vi "Write Element of Exp Groups.vi"(8 "error in (no error)":errorcluster, 9 "Experiments_group.lvclass":refnum<class "Experiments_group.lvclass">, 10 "index":i32=-1, 11 "Control-Client in":refnum<class "Control-Client.lvclass">) -> (0 "error out":errorcluster, 3 "Control-Client out":refnum<class "Control-Client.lvclass">)   [LabVIEW 2018, in "Control-Client.lvclass"]
uses:
  Control-Client.lvclass
  Experiments/Experiments_group.lvclass
  Control-Client.lvclass/Control-Client.ctl
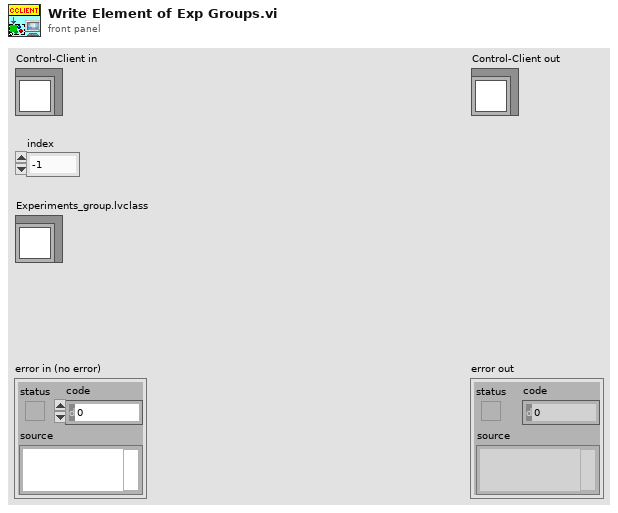
[diagram p1: front panel]
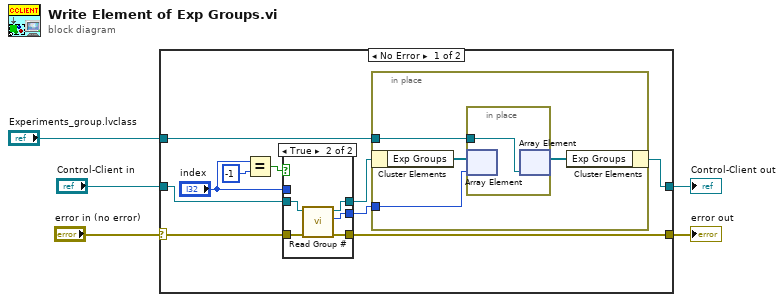
[diagram p0: block diagram]
diagram:
  n1 = case shown="No Error" "error in (no error)" {
    selector: "error in (no error)" -> [w11 w29]
    tunnel: [w12 w29] -> w4
    tunnel: [w7 w30] -> w2
    tunnel: "Control-Client in" -> [w10 w30]
    tunnel: "Experiments_group.lvclass" -> [w8 _]
    frame No Error {
      n2 = Equal?(x="index", y=-1) -> (x = y?=w14:bool)
      n3 = case shown="True" w14 {
        tunnel: [w23 w28] -> w9
        tunnel: "index" -> [w23 _]
        tunnel: [w22 w27] -> w12
        tunnel: w11 -> [w22 w26]
        tunnel: w10 -> [w21 w25]
        tunnel: [w21 w24] -> w6
        frame False {
        }
        frame True {
          n4 = call "Read Group #.vi"("error in (no error)"=w26, "Control-Client in"=w25) -> ("error out"=w27:errorcluster, "Group #"=w28:i32, "Control-Client out"=w24:refnum<class "Control-Client.lvclass">)  [unwired: 7 in]
        }
      }
      n5 = in-place {
        in-place-border: w9 -> [w18]
        in-place-border: w8 -> [w16]
        n6 = in-place-cluster #1(w6) -> ("Exp Groups"=w19:refnum<class "Experiments_group.lvclass">[])
        n7 = in-place {
          in-place-border: w16 -> [w20]
          n8 = in-place-array #2(w19, w18) -> ()  [unwired: 1 out]
          n9 = in-place-array #2(w20) -> (w17:refnum<class "Experiments_group.lvclass">[])  [unwired: 1 out]
        }
        n10 = in-place-cluster #1("Exp Groups"=w17) -> (w7:refnum<class "Control-Client.lvclass">)
      }
    }
    frame Error {
    }
  }
  "error out" <- w4
  "Control-Client out" <- w2
